vi "글로벌 1.vi"() -> ()   [LabVIEW 2017]
panel:
  in  "문자열":string
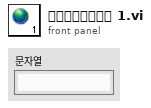
[diagram p1: front panel]
diagram:
